vi "_Calculate spacing.vi"(2 "Button Size":cluster{"Width":i32, "Height":i32}, 3 "Icon Size":cluster{"Width":i32, "Height":i32}, 4 "Text Size":cluster{"Width":i16, "Height":i16}) -> (0 "Vert. spacing":i32, 1 "Horiz. spacing":i32)   [LabVIEW 2012]
doc: "Calculates the spacing, given text size, icon size and button size."
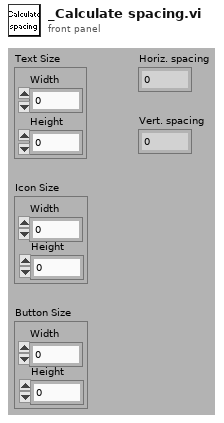
[diagram p1: front panel]
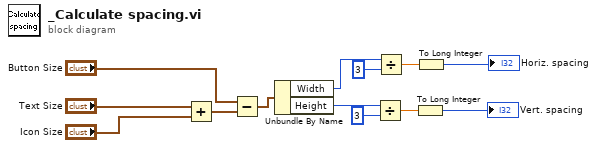
[diagram p0: block diagram]
diagram:
  n1 = Add(x="Text Size", y="Icon Size") -> (x+y=w4:cluster{"Width":i32, "Height":i32})
  n2 = Subtract(x="Button Size", y=w4) -> (x-y=w6:cluster{"Width":i32, "Height":i32})
  n3 = Unbundle By Name(w6) -> ("Width"=w12:i32, "Height"=w7:i32)
  n4 = Divide(x=w7, y=3) -> (x/y=w9:dbl)
  n5 = Divide(x=w12, y=3) -> (x/y=w10:dbl)
  n6 = To Long Integer(number=w9) -> (32bit integer=→"Vert. spacing":i32)
  n7 = To Long Integer(number=w10) -> (32bit integer=→"Horiz. spacing":i32)
